vi "Func-엑셀 데이터를 그래프로 출력.vi"() -> ()   [LabVIEW 2015] (continued)
39.607\n25\t24.51\t39.603\n25\t24.51\t39.598\n25\t24.51\t39.589\n25\t24.51\t39.584\n25\t24.51\t39.573\n25\t24.51\t39.569\n25\t24.51\t39.561\n25\t24.51\t39.55\n25\t24.52\t39.547\n25\t24.52\t39.539\n25\t24.52\t39.529\n25\t24.52\t39.52\n25\t24.52\t39.513\n25\t24.53\t39.501\n25\t24.53\t39.496\n25\t24.53\t39.49\n25\t24.53\t39.486\n25\t24.53\t39.48\n25\t24.53\t39.476\n25\t24.53\t39.473\n25\t24.53\t39.465\n25\t24.53\t39.455\n25\t24.53\t39.442\n25\t24.53\t39.437\n25\t24.53\t39.427\n25\t24.53\t39.411\n25\t24.53\t39.404\n25\t24.53\t39.397\n25\t24.53\t39.392\n25\t24.54\t39.384\n25\t24.54\t39.377\n25\t24.54\t39.373\n25\t24.54\t39.365\n25\t24.54\t39.359\n25\t24.54\t39.35\n25\t24.54\t39.344\n25\t24.54\t39.332\n25\t24.54\t39.327\n25\t24.55\t39.323\n25\t24.55\t39.314\n25\t24.55\t39.304\n25\t24.55\t39.298\n25\t24.56\t39.291\n25\t24.56\t39.289\n25\t24.56\t39.282\n25\t24.56\t39.276\n25\t24.57\t39.275\n25\t24.57\t39.268\n25\t24.57\t39.263\n25\t24.57\t39.252\n25\t24.57\t39.247\n25\t24.57\t39.238\n25\t24.57\t39.225\n25\t24.58\t39.219\n25\t24.58\t39.207\n25\t24.58\t39.201\n25\t24.58\t39.195\n25\t24.58\t39.186\n25\t24.58\t39.182\n25\t24.59\t39.174\n25\t24.59\t39.166\n25\t24.59\t39.156\n25\t24.59\t39.141\n25\t24.59\t39.132\n25\t24.6\t39.124\n25\t24.6\t39.115\n25\t24.6\t39.106\n25\t24.6\t39.1\n25\t24.6\t39.094\n25\t24.6\t39.089\n25\t24.6\t39.085\n25\t24.6\t39.077\n25\t24.6\t39.071\n25\t24.61\t39.07\n25\t24.61\t39.062\n25\t24.62\t39.056\n25\t24.62\t39.048\n25\t24.62\t39.041\n25\t24.62\t39.036\n25\t24.62\t39.026\n25\t24.62\t39.017\n25\t24.62\t39.009\n25\t24.62\t39.001\n25\t24.62\t38.99\n25\t24.62\t38.983\n25\t24.62\t38.979\n25\t24.63\t38.971\n25\t24.63\t38.963\n25\t24.63\t38.96\n25\t24.63\t38.953\n25\t24.63\t38.946\n25\t24.63\t38.942\n25\t24.63\t38.932\n25\t24.64\t38.927\n25\t24.64\t38.918\n25\t24.64\t38.909\n25\t24.64\t38.898\n25\t24.64\t38.889\n25\t24.65\t38.884\n25\t24.65\t38.877\n25\t24.65\t38.873\n25\t24.65\t38.862\n25\t24.65\t38.86\n25\t24.65\t38.851\n25\t24.65\t38.842\n25\t24.66\t38.837\n25\t24.66\t38.832\n25\t24.66\t38.829\n25\t24.66\t38.823\n25\t24.66\t38.808\n25\t24.66\t38.799\n25\t24.66\t38.791\n25\t24.67\t38.776\n25\t24.67\t38.764\n25\t24.67\t38.757\n25\t24.68\t38.75\n25\t24.68\t38.746\n25\t24.68\t38.737\n25\t24.68\t38.731\n25\t24.68\t38.727\n25\t24.68\t38.719\n25\t24.69\t38.712\n25\t24.69\t38.707\n25\t24.69\t38.703\n25\t24.69\t38.696\n25\t24.7\t38.689\n25\t24.69\t38.685\n25\t24.7\t38.683\n25\t24.7\t38.675\n25\t24.7\t38.668\n25\t24.71\t38.66\n25\t24.71\t38.656\n25\t24.71\t38.648\n25\t24.71\t38.635\n25\t24.71\t38.63\n25\t24.71\t38.625\n25\t24.71\t38.615\n25\t24.71\t38.608\n25\t24.71\t38.598\n25\t24.72\t38.594\n25\t24.72\t38.584\n25\t24.72\t38.579\n25\t24.72\t38.571\n25\t24.73\t38.562\n25\t24.73\t38.556\n25\t24.73\t38.548\n25\t24.73\t38.543\n25\t24.73\t38.532\n25\t24.73\t38.523\n25\t24.74\t38.523\n25\t24.74\t38.514\n25\t24.74\t38.508\n25\t24.75\t38.502\n25\t24.75\t38.495\n25\t24.75\t38.489\n25\t24.75\t38.478\n25\t24.75\t38.469\n25\t24.75\t38.465\n25\t24.75\t38.461\n25\t24.76\t38.454\n25\t24.76\t38.448\n25\t24.76\t38.441\n25\t24.76\t38.434\n25\t24.76\t38.428\n25\t24.76\t38.422\n25\t24.76\t38.414\n25\t24.77\t38.406\n25\t24.77\t38.405\n25\t24.77\t38.393\n25\t24.77\t38.386\n25\t24.77\t38.377\n25\t24.77\t38.368\n25\t24.77\t38.362\n25\t24.78\t38.35\n25\t24.78\t38.345\n25\t24.77\t38.339\n25\t24.78\t38.334\n25\t24.78\t38.327\n25\t24.78\t38.327\n25\t24.78\t38.32\n25\t24.78\t38.314\n25\t24.78\t38.308\n25\t24.79\t38.301\n25\t24.78\t38.295\n25\t24.79\t38.288\n25\t24.79\t38.286\n25\t24.79\t38.281\n25\t24.79\t38.271\n25\t24.8\t38.258\n25\t24.79\t38.25\n25\t24.79\t38.241\n25\t24.79\t38.228\n25\t24.8\t38.216\n25\t24.8\t38.213\n25\t24.8\t38.206\n25\t24.8\t38.201\n25\t24.8\t38.194\n25\t24.8\t38.185\n25\t24.8\t38.18\n25\t24.8\t38.175\n25\t24.8\t38.164\n25\t24.8\t38.159\n25\t24.81\t38.16\n25\t24.81\t38.154\n25\t24.81\t38.148\n25\t24.81\t38.137\n25\t24.81\t38.135\n25\t24.81\t38.129\n25\t24.81\t38.118\n25\t24.81\t38.114\n25\t24.81\t38.112\n25\t24.82\t38.111\n25\t24.82\t38.101\n25\t24.82\t38.096\n25\t24.82\t38.091\n25\t24.83\t38.081\n25\t24.83\t38.07\n25\t24.83\t38.06\n25\t24.83\t38.054\n25\t24.83\t38.047\n25\t24.83\t38.037\n25\t24.83\t38.029\n25\t24.83\t38.025\n25\t24.83\t38.02\n25\t24.83\t38.013\n25\t24.83\t38.004\n25\t24.83\t37.995\n25\t24.83\t37.996\n25\t24.84\t37.989\n25\t24.84\t37.984\n25\t24.84\t37.979\n25\t24.84\t37.975\n25\t24.84\t37.968\n25\t24.84\t37.96\n25\t24.84\t37.955\n25\t24.84\t37.946\n25\t24.84\t37.941\n25\t24.84\t37.937\n25\t24.85\t37.931\n25\t24.86\t37.925\n25\t24.87\t37.917\n25\t24.88\t37.907\n25\t24.89\t37.899\n25\t24.9\t37.892\n25\t24.91\t37.881\n25\t24.92\t37.876\n25\t24.93\t37.87\n25\t24.94\t37.862\n25\t24.95\t37.858\n25\t24.96\t37.853\n25\t24.97\t37.846\n25\t24.98\t37.836\n25\t25\t37.832\n25\t24.96\t37.823\n25\t24.96\t37.817\n25\t24.96\t37.809\n25\t24.96\t37.797\n25\t24.96\t37.796\n25\t24.96\t37.789\n25\t24.97\t37.784\n25\t24.97\t37.781\n25\t24.97\t37.777\n25\t24.97\t37.771\n25\t24.97\t37.759\n25\t24.97\t37.752\n25\t24.97\t37.748\n25\t24.97\t37.741\n25\t24.97\t37.736\n25\t24.97\t37.732\n25\t24.97\t37.73\n25\t24.97\t37.72\n25\t24.97\t37.715\n25\t24.97\t37.71\n25\t24.97\t37.701\n25\t24.97\t37.694\n25\t24.97\t37.689\n25\t24.97\t37.684\n25\t24.97\t37.678\n25\t24.97\t37.67\n25\t24.97\t37.665\n25\t24.97\t37.66\n25\t24.97\t37.653\n25\t24.97\t37.641\n25\t24.97\t37.632\n25\t24.97\t37.627\n25\t24.97\t37.616\n25\t24.97\t37.611\n25\t24.97\t37.607\n25\t24.97\t37.603\n25\t24.97\t37.603\n25\t24.97\t37.596\n25\t24.97\t37.588\n25\t24.97\t37.586\n25\t24.97\t37.579\n25\t24.97\t37.575\n25\t24.97\t37.568\n25\t24.97\t37.561\n25\t24.97\t37.561\n25\t24.97\t37.554\n25\t24.97\t37.545\n25\t24.97\t37.537\n25\t24.97\t37.528\n25\t24.97\t37.522\n25\t24.97\t37.515\n25\t24.97\t37.505\n25\t24.97\t37.498\n25\t24.97\t37.491\n25\t24.97\t37.488\n25\t24.97\t37.481\n25\t24.97\t37.476\n25\t24.97\t37.471\n25\t24.97\t37.464\n25\t24.97\t37.458\n25\t24.97\t37.455\n25\t24.97\t37.445\n25\t24.97\t37.439\n25\t24.97\t37.435\n25\t24.97\t37.428\n25\t24.97\t37.423\n25\t24.97\t37.416\n25\t24.97\t37.413\n25\t24.97\t37.405\n25\t24.97\t37.401\n25\t24.97\t37.396\n25\t24.98\t37.391\n25\t24.98\t37.388\n25\t24.98\t37.375\n25\t24.98\t37.371\n25\t24.98\t37.366\n25\t24.98\t37.359\n25\t24.98\t37.351\n25\t24.98\t37.345\n25\t24.98\t37.341\n25\t24.98\t37.336\n25\t24.98\t37.329\n25\t24.98\t37.318\n25\t24.98\t37.312\n25\t24.98\t37.301\n25\t24.98\t37.297\n25\t24.98\t37.291\n25\t24.98\t37.282\n25\t24.98\t37.276\n25\t24.98\t37.271\n25\t24.98\t37.268\n25\t24.98\t37.26\n25\t24.98\t37.256\n25\t24.98\t37.252\n25\t24.98\t37.251\n25\t24.98\t37.248\n25\t24.98\t37.24\n25\t24.98\t37.236\n25\t24.98\t37.23\n25\t24.98\t37.226\n25\t24.98\t37.222\n25\t24.98\t37.214\n25\t24.98\t37.207\n25\t24.98\t37.203\n25\t24.98\t37.197\n25\t24.98\t37.186\n25\t24.98\t37.179\n25\t24.98\t37.172\n25\t24.98\t37.166\n25\t24.98\t37.161\n25\t24.98\t37.155\n25\t24.98\t37.148\n25\t24.98\t37.142\n25\t24.98\t37.143\n25\t24.98\t37.136\n25\t24.98\t37.132\n25\t24.98\t37.125\n25\t24.98\t37.119\n25\t24.98\t37.114\n25\t24.98\t37.109\n25\t24.98\t37.105\n25\t24.98\t37.1\n25\t24.98\t37.096\n25\t24.98\t37.09\n25\t24.98\t37.085\n25\t24.98\t37.074\n25\t24.98\t37.063\n25\t24.98\t37.056\n25\t24.98\t37.047\n25\t24.98\t37.043\n25\t24.98\t37.035\n25\t24.98\t37.028\n25\t24.98\t37.026\n25\t24.98\t37.024\n25\t24.98\t37.021\n25\t24.98\t37.017\n25\t24.98\t37.016\n25\t24.98\t37.008\n25\t24.98\t37.005\n25\t24.98\t37.001\n25\t24.98\t36.993\n25\t24.98\t36.991\n25\t24.98\t36.985\n25\t25\t36.98\n25\t25\t36.974\n25\t25\t36.968\n25\t25\t36.957\n25\t25\t36.947\n25\t25\t36.939\n25\t25\t36.935\n25\t24.98\t36.931\n25\t25\t36.927\n25\t25\t36.923\n25\t25\t36.919\n25\t25\t36.912\n25\t25\t36.904\n25\t25\t36.901\n25\t25\t36.895\n25\t25\t36.891\n25\t25\t36.885\n25\t24.98\t36.88\n25\t24.98\t36.873\n25\t24.98\t36.87\n25\t25\t36.865\n25\t25\t36.857\n25\t25\t36.856\n25\t25\t36.852\n25\t25\t36.846\n25\t25\t36.838\n25\t25\t36.832\n25\t25\t36.825\n25\t25\t36.82\n25\t25\t36.816\n25\t24.98\t36.812\n25\t24.98\t36.809\n25\t24.98\t36.798\n25\t24.98\t36.796\n25\t24.98\t36.791\n25\t25\t36.784\n25\t25\t36.78\n25\t25\t36.774\n25\t25\t36.77\n25\t25\t36.762\n25\t25\t36.759\n25\t25\t36.752\n25\t25\t36.746\n25\t25\t36.738\n25\t25\t36.732\n25\t25\t36.729\n25\t25\t36.721\n25\t25\t36.713\n25\t25\t36.711\n25\t25\t36.711\n25\t25\t36.705\n25\t25\t36.706\n25\t25\t36.704\n25\t25\t36.699\n25\t25\t36.695\n25\t25\t36.687\n25\t25\t36.684\n25\t25\t36.676\n25\t25\t36.671\n25\t25\t36.668\n25\t25\t36.663\n25\t25\t36.656\n25\t25\t36.648\n25\t25\t36.645\n25\t25\t36.637\n25\t25\t36.63\n25\t25\t36.624\n25\t25\t36.612\n25\t25\t36.612\n25\t25\t36.607\n25\t25\t36.6\n25\t25\t36.595\n25\t25\t36.591\n25\t25\t36.591\n25\t25\t36.583\n25\t25\t36.575\n25\t25\t36.569\n25\t25\t36.567\n25\t25\t36.562\n25\t25\t36.554\n25\t25\t36.549\n25\t25\t36.545\n25\t25\t36.541\n25\t25\t36.536\n25\t25\t36.533\n25\t25\t36.525\n25\t25\t36.523\n25\t25\t36.517\n25\t25\t36.516\n25\t25\t36.51\n25\t25\t36.506\n25\t25\t36.507\n25\t25\t36.505\n25\t25\t36.498\n25\t25\t36.493\n25\t25\t36.489\n25\t25\t36.48\n25\t25\t36.473\n25\t25\t36.466\n25\t25\t36.462\n25\t25\t36.456\n25\t25\t36.454\n25\t25\t36.449\n25\t25\t36.442\n25\t25\t36.44\n25\t25\t36.431\n25\t25\t36.425\n25\t25\t36.418\n25\t25\t36.412\n25\t25\t36.409\n25\t25\t36.404\n25\t25\t36.398\n25\t25\t36.397\n25\t25\t36.398\n25\t25\t36.391\n25\t25\t36.391\n25\t25\t36.384\n25\t25\t36.377\n25\t25\t36.37\n25\t25\t36.365\n25\t25\t36.362\n25\t25\t36.355\n25\t25\t36.352\n25\t25\t36.349\n25\t25\t36.347\n25\t25\t36.34\n25\t25\t36.33\n25\t25\t36.326\n25\t25\t36.322\n25\t25\t36.314\n25\t25\t36.306\n25\t25\t36.298\n25\t25\t36.295\n25\t25\t36.287\n25\t25\t36.284\n25\t25\t36.28\n25\t25\t36.279\n25\t25\t36.276\n25\t25\t36.271\n25\t25\t36.268\n25\t25\t36.262\n25\t25\t36.259\n25\t25\t36.254\n25\t25\t36.246\n25\t25\t36.244\n25\t25\t36.241\n25\t25\t36.237\n25\t25\t36.233\n25\t25\t36.226\n25\t25\t36.22\n25\t25\t36.216\n25\t25\t36.211\n25\t25\t36.203\n25\t25\t36.198\n25\t25\t36.196\n25\t25\t36.193\n25\t25\t36.187\n25\t25\t36.182\n25\t25\t36.178\n25\t25\t36.175\n25\t25\t36.171\n25\t25\t36.166\n25\t25\t36.163\n25\t25\t36.159\n25\t25\t36.152\n25\t25\t36.15\n25\t25\t36.141\n25\t25\t36.138\n25\t25\t36.134\n25\t25\t36.13\n25\t25\t36.124\n25\t25\t36.119\n25\t25\t36.116\n25\t25\t36.113\n25\t25\t36.11\n25\t25\t36.105\n25\t25\t36.104\n25\t25\t36.099\n25\t25\t36.093\n25\t25\t36.087\n25\t25\t36.08\n25\t25\t36.075\n25\t25\t36.07\n25\t25\t36.066\n25\t25\t36.064\n25\t25\t36.062\n25\t25\t36.063\n25\t25\t36.058\n25\t25\t36.059\n25\t25\t36.048\n25\t25\t36.042\n25\t25\t36.037\n25\t25\t36.028\n25\t25\t36.027\n25\t25\t36.022\n25\t25\t36.019\n25\t25\t36.015\n25\t25\t36.013\n25\t25\t36.008\n25\t25\t35.999\n25\t25\t35.995\n25\t25\t35.992\n25\t25\t35.987\n25\t25\t35.984\n25\t25\t35.979\n25\t25\t35.977\n25\t25\t35.972\n25\t25\t35.964\n25\t25\t35.961\n25\t25\t35.957\n25\t25\t35.948\n25\t25\t35.945\n25\t25\t35.94\n25\t25\t35.939\n25\t25\t35.935\n25\t25\t35.931\n25\t25\t35.93\n25\t25\t35.928\n25\t25\t35.924\n25\t25\t35.917\n25\t25\t35.914\n25\t25\t35.908\n25\t25\t35.906\n25\t25\t35.896\n25\t25\t35.896\n25\t25\t35.891\n25\t25\t35.886\n25\t25\t35.881\n25\t25\t35.872\n25\t25\t35.872\n25\t25\t35.866\n25\t25\t35.864\n25\t25\t35.861\n25\t25\t35.86\n25\t25\t35.862\n25\t25\t35.855\n25\t25\t35.848\n25\t25\t35.839\n25\t25\t35.834\n25\t25\t35.824\n25\t25\t35.819\n25\t25\t35.818\n25\t25\t35.817\n25\t25\t35.814\n25\t25\t35.812\n25\t25\t35.807\n25\t25\t35.801\n25\t25\t35.796\n25\t25\t35.789\n25\t25\t35.786\n25\t25\t35.781\n25\t25\t35.776\n25\t25\t35.772\n25\t25\t35.768\n25\t25\t35.763\n25\t25\t35.754\n25\t25\t35.75\n25\t25\t35.745\n25\t25\t35.741\n25\t25\t35.737\n25\t25\t35.735\n25\t25\t35.739\n25\t25\t35.738\n25\t25\t35.733\n25\t25\t35.73\n25\t25\t35.727\n25\t25\t35.722\n25\t25\t35.714\n25\t25\t35.709\n25\t25\t35.709\n25\t25\t35.702\n25\t25\t35.698\n25\t25\t35.693\n25\t25\t35.689\n25\t25\t35.684\n25\t25\t35.677\n25\t25\t35.676\n25\t25\t35.673\n25\t25\t35.668\n25\t25\t35.666\n25\t25\t35.661\n25\t25\t35.659\n25\t25\t35.654\n25\t25\t35.648\n25\t25\t35.647\n25\t25\t35.644\n25\t25\t35.641\n25\t25\t35.638\n25\t25\t35.635\n25\t25\t35.632\n25\t25\t35.629\n25\t25\t35.623\n25\t25\t35.619\n25\t25\t35.612\n25\t25\t35.609\n25\t25\t35.604\n25\t25\t35.599\n25\t25\t35.597\n25\t25\t35.59\n25\t25\t35.592\n25\t25\t35.59\n25\t25\t35.584\n25\t25\t35.584\n25\t25\t35.581\n25\t25\t35.58\n25\t25\t35.576\n25\t25\t35.57\n25\t25\t35.566\n25\t25\t35.562\n25\t25\t35.552\n25\t25\t35.549\n25\t25\t35.544\n25\t25\t35.539\n25\t25\t35.535\n25\t25\t35.531\n25\t25\t35.531\n25\t25\t35.527\n25\t25\t35.523\n25\t25\t35.52\n25\t25\t35.518\n25\t25\t35.513\n25\t25\t35.508\n25\t25\t35.5\n25\t25\t35.498\n25\t25\t35.494\n25\t25\t35.49\n25\t25\t35.491\n25\t25\t35.482\n25\t25\t35.481\n25\t25\t35.477\n25\t25\t35.472\n25\t25\t35.465\n25\t25\t35.461\n25\t25\t35.461\n25\t25\t35.459\n25\t25\t35.452\n25\t25\t35.446\n25\t25\t35.451\n25\t25\t35.447\n25\t25\t35.443\n25\t25\t35.44\n25\t25\t35.442\n25\t25\t35.44\n25\t25\t35.432\n25\t25\t35.425\n25\t25\t35.419\n25\t25\t35.415\n25\t25\t35.409\n25\t25\t35.405\n25\t25\t35.403\n25\t25\t35.407\n25\t25\t35.403\n25\t25\t35.396\n25\t25\t35.393\n25\t25\t35.392\n25\t25\t35.389\n25\t25\t35.377\n25\t25\t35.378\n25\t25\t35.38\n25\t25\t35.375\n25\t25\t35.371\n25\t25\t35.369\n25\t25\t35.366\n25\t25\t35.362\n25\t25\t35.359\n25\t25\t35.354\n25\t25\t35.348\n25\t25\t35.345\n25\t25\t35.345\n25\t25\t35.343\n25\t25\t35.34\n25\t25\t35.338\n25\t25\t35.334\n25\t25\t35.33\n25\t25\t35.321\n25\t25\t35.314\n25\t25\t35.314\n25\t25\t35.305\n25\t25\t35.305\n25\t25\t35.304\n25\t25\t35.302\n25\t25\t35.299\n25\t25\t35.294\n25\t25\t35.287\n25\t25\t35.281\n25\t25\t35.277\n25\t25\t35.27\n25\t25\t35.268\n25\t25\t35.264\n25\t25\t35.263\n25\t25\t35.26\n25\t25\t35.255\n25\t25\t35.251\n25\t25\t35.248\n25\t25\t35.242\n25\t25\t35.243\n25\t25\t35.242\n25\t25\t35.239\n25\t25\t35.239\n25\t25\t35.235\n25\t25\t35.233\n25\t25\t35.227\n25\t25\t35.225\n25\t25\t35.221\n25\t25\t35.218\n25\t25\t35.214\n25\t25\t35.209\n25\t25\t35.205\n25\t25\t35.199\n25\t25\t35.196\n25\t25\t35.193\n25\t25\t35.193\n25\t25\t35.184\n25\t25\t35.185\n25\t25\t35.18\n25\t25\t35.173\n25\t25\t35.172\n25\t25\t35.164\n25\t25\t35.16\n25\t25\t35.153\n25\t25\t35.15\n25\t25\t35.148\n25\t25\t35.143\n25\t25\t35.146\n25\t25\t35.147\n25\t25\t35.144\n25\t25\t35.14\n25\t25\t35.138\n25\t25\t35.138\n25\t25\t35.131\n25\t25\t35.127\n25\t25\t35.125\n25\t25\t35.12\n25\t25\t35.12\n25\t25\t35.117\n25\t25\t35.111\n25\t25\t35.106\n25\t25\t35.104\n25\t25\t35.102\n25\t25\t35.098\n25\t25\t35.093\n25\t25\t35.093\n25\t25\t35.089\n25\t25\t35.086\n25\t25\t35.083\n25\t25\t35.078\n25\t25\t35.074\n25\t25\t35.073\n25\t25\t35.069\n25\t25\t35.068\n25\t25\t35.064\n25\t25\t35.063\n25\t25\t35.062\n25\t25\t35.054\n25\t25\t35.052\n25\t25\t35.05\n25\t25\t35.042\n25\t25\t35.037\n25\t25\t35.034\n25\t25\t35.027\n25\t25\t35.026\n25\t25\t35.018\n25\t25\t35.017\n25\t25\t35.014\n25\t25\t35.009\n25\t25\t35.007\n25\t25\t35.005\n25\t25\t35.005\n25\t25\t35.004\n25\t25\t35.005\n25\t25\t35.002\n25\t25\t35\n25\t25\t34.996\n25\t25\t34.989\n25\t25\t34.982\n25\t25\t34.977\n25\t25\t34.975\n25\t25\t34.972\n25\t25\t34.968\n25\t25\t34.97\n25\t25\t34.965\n25\t25\t34.964\n25\t25\t34.962\n25\t25\t34.961\n25\t25\t34.961\n25\t25\t34.954\n25\t25\t34.955\n25\t25\t34.95\n25\t25\t34.945\n25\t25\t34.943\n25\t25\t34.941\n25\t25\t34.936\n25\t25\t34.932\n25\t25\t34.931\n25\t25\t34.93\n25\t25\t34.931\n25\t25\t34.928\n25\t25\t34.927\n25\t25\t34.925\n25\t25\t34.921\n25\t25\t34.917\n25\t25\t34.911\n25\t25\t34.904\n25\t25\t34.902\n25\t25\t34.898\n25\t25\t34.895\n25\t25\t34.895\n25\t25\t34.893\n25\t25\t34.888\n25\t25\t34.888\n25\t25\t34.884\n25\t25\t34.876\n25\t25\t34.871\n25\t25\t34.868\n25\t25\t34.867\n25\t25\t34.862\n25\t25\t34.86\n25\t25\t34.861\n25\t25\t34.857\n25\t25\t34.855\n25\t25\t34.848\n25\t25\t34.845\n25\t25\t34.847\n25\t25\t34.839\n25\t25\t34.838\n25\t25\t34.835\n25\t25\t34.836\n25\t25\t34.831\n25\t25\t34.827\n25\t25\t34.825\n25\t25\t34.823\n25\t25\t34.823\n25\t25\t34.815\n25\t25\t34.812\n25\t25\t34.807\n25\t25\t34.805\n25\t25\t34.799\n25\t25\t34.793\n25\t25\t34.791\n25\t25\t34.789\n25\t25\t34.789\n25\t25\t34.784\n25\t25\t34.786\n25\t25\t34.786\n25\t25\t34.781\n25\t25\t34.779\n25\t25\t34.774\n25\t25\t34.775\n25\t25\t34.772\n25\t25\t34.766\n25\t25\t34.766\n25\t25\t34.767\n25\t25\t34.766\n25\t25\t34.763\n25\t25\t34.758\n25\t25\t34.755\n25\t25\t34.754\n25\t25\t34.747\n25\t25\t34.737\n25\t25\t34.734\n25\t25\t34.731\n25\t25\t34.725\n25\t25\t34.721\n25\t25\t34.719\n25\t25\t34.716\n25\t25\t34.713\n25\t25\t34.71\n25\t25\t34.707\n25\t25\t34.704\n25\t25\t34.701\n25\t25\t34.701\n25\t25\t34.695\n25\t25\t34.696\n25\t25\t34.695\n25\t25\t34.693\n25\t25\t34.688\n25\t25\t34.683\n25\t25\t34.686\n25\t25\t34.682\n25\t25\t34.68\n25\t25\t34.679\n25\t25\t34.676\n25\t25\t34.675\n25\t25\t34.675\n25\t25\t34.671\n25\t25\t34.667\n25\t25\t34.665\n25\t25\t34.662\n25\t25\t34.654\n25\t25\t34.649\n25\t25\t34.646\n25\t25\t34.645\n25\t25\t34.642\n25\t25\t34.636\n25\t25\t34.638\n25\t25\t34.636\n25\t25\t34.633\n25\t25\t34.627\n25\t25\t34.626\n25\t25\t34.626\n25\t25\t34.625\n25\t25\t34.623\n25\t25\t34.618\n25\t25\t34.614\n25\t25\t34.611\n25\t25\t34.608\n25\t25\t34.607\n25\t25\t34.6\n25\t25\t34.6\n25\t25\t34.598\n25\t25\t34.596\n25\t25\t34.594\n25\t25\t34.588\n25\t25\t34.591\n25\t25\t34.589\n25\t25\t34.586\n25\t25\t34.583\n25\t25\t34.584\n25\t25\t34.582\n25\t25\t34.575\n25\t25\t34.572\n25\t25\t34.573\n25\t25\t34.568\n25\t25\t34.564\n25\t25\t34.563\n25\t25\t34.562\n25\t25\t34.558\n25\t25\t34.554\n25\t25\t34.551\n25\t25\t34.545\n25\t25\t34.541\n25\t25\t34.541\n25\t25\t34.541\n25\t25\t34.541\n25\t25\t34.537\n25\t25\t34.536\n25\t25\t34.536\n25\t25\t34.533\n25\t25\t34.531\n25\t25\t34.526\n25\t25\t34.523\n25\t25\t34.524\n25\t25\t34.52\n25\t25\t34.514\n25\t25\t34.511\n25\t25\t34.508\n25\t25\t34.507\n25\t25\t34.502\n25\t25\t34.498\n25\t25\t34.496\n25\t25\t34.495\n25\t25\t34.495\n25\t25\t34.492\n25\t25\t34.49\n25\t25\t34.491\n25\t25\t34.49\n25\t25\t34.487\n25\t25\t34.484\n25\t25\t34.481\n25\t25\t34.482\n25\t25\t34.479\n25\t25\t34.47\n25\t25\t34.466\n25\t25\t34.461\n25\t25\t34.455\n25\t25\t34.45\n25\t25\t34.446\n25\t25\t34.447\n25\t25\t34.445\n25\t25\t34.439\n25\t25\t34.444\n25\t25\t34.443\n25\t25\t34.442\n25\t25\t34.439\n25\t25\t34.438\n25\t25\t34.438\n25\t25\t34.435\n25\t25\t34.432\n25\t25\t34.43\n25\t25\t34.428\n25\t25\t34.425\n25\t25\t34.427\n25\t25\t34.423\n25\t25\t34.423\n25\t25\t34.421\n25\t25\t34.42\n25\t25\t34.414\n25\t25\t34.41\n25\t25\t34.407\n25\t25\t34.402\n25\t25\t34.398\n25\t25\t34.396\n25\t25\t34.395\n25\t25\t34.389\n25\t25\t34.388\n25\t25\t34.386\n25\t25\t34.383\n25\t25\t34.379\n25\t25\t34.378\n25\t25\t34.376\n25\t25\t34.372\n25\t25\t34.37\n25\t25\t34.368\n25\t25\t34.367\n25\t25\t34.364\n25\t25\t34.361\n25\t25\t34.359\n25\t25\t34.359\n25\t25\t34.358\n25\t25\t34.354\n25\t25\t34.348\n25\t25\t34.346\n25\t25\t34.349\n25\t25\t34.346\n25\t25\t34.341\n25\t25\t34.341\n25\t25\t34.343\n25\t25\t34.341\n25\t25\t34.334\n25\t25\t34.329\n25\t25\t34.328\n25\t25\t34.326\n25\t25\t34.32\n25\t25\t34.319\n25\t25\t34.321\n25\t25\t34.32\n25\t25\t34.319\n25\t25\t34.313\n25\t25\t34.309\n25\t25\t34.309\n25\t25\t34.305\n25\t25\t34.301\n25\t25\t34.299\n25\t25\t34.298\n25\t25\t34.304\n25\t25\t34.296\n25\t25\t34.291\n25\t25\t34.287\n25\t25\t34.282\n25\t25\t34.279\n25\t25\t34.274\n25\t25\t34.273\n25\t25\t34.274\n25\t25\t34.277\n25\t25\t34.278\n25\t25\t34.277\n25\t25\t34.273\n25\t25\t34.273\n25\t25\t34.27\n25\t25\t34.268\n25\t25\t34.263\n25\t25\t34.262\n25\t25\t34.263\n25\t25\t34.261\n25\t25\t34.254\n25\t25\t34.25\n25\t25\t34.247\n25\t25\t34.243\n25\t25\t34.238\n25\t25\t34.236\n25\t25\t34.236\n25\t25\t34.235\n25\t25\t34.235\n25\t25\t34.232\n25\t25\t34.232\n25\t25\t34.23\n25\t25\t34.23\n25\t25\t34.226\n25\t25\t34.223\n25\t25\t34.219\n25\t25\t34.218\n25\t25\t34.218\n25\t25\t34.214\n25\t25\t34.212\n25\t25\t34.21\n25\t25\t34.208\n25\t25\t34.202\n25\t25\t34.198\n25\t25\t34.198\n25\t25\t34.197\n25\t25\t34.197\n25\t25\t34.195\n25\t25\t34.195\n25\t25\t34.193\n25\t25\t34.193\n25\t25\t34.191\n25\t
